vi "Handle Brushed Speed.vi"(9 "Brushless":bool, 11 "Tank Data IN":dbl[](array[numeric])) -> (3 "Tank Data OUT":dbl[](array[numeric]))   [LabVIEW 2013]
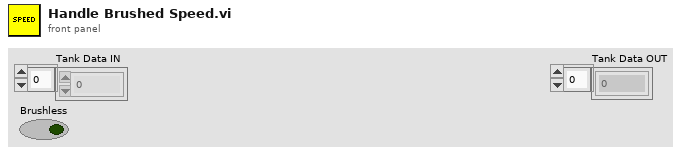
[diagram p1: front panel]
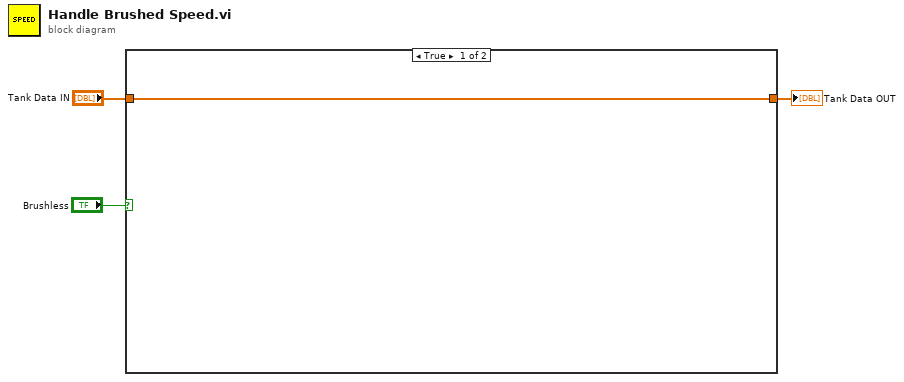
[diagram p0: block diagram]
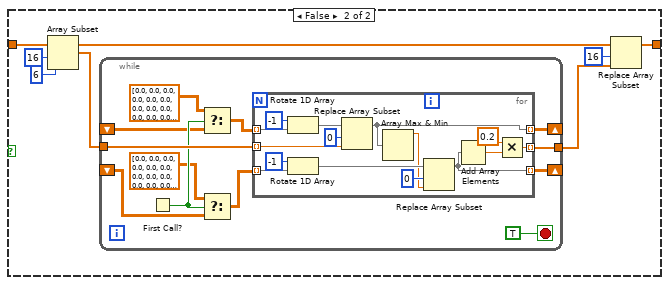
[diagram p2: hidden frame]
diagram:
  n1 = case shown="True" "Brushless" {
    tunnel: "Tank Data IN" -> [w4 w9]
    tunnel: [w4 w8] -> w2
    frame True {
    }
    frame False {
      n2 = Array Subset(array=w9, index=16, length=6 ("index")) -> (w5:dbl[])
      n3 = while {
        tunnel: [w22] -> w6
        shift-right: [w23] -> _
        shift-left: _ -> [w16]
        tunnel: w5 -> [w20]
        shift-right: [w21] -> _
        shift-left: _ -> [w17]
        stop <- TRUE stop-if-true
        n4 = First Call?() -> (First Call?: T/F=w18:bool)
        n5 = Select(t=dbl[][] [[0.0, 0.0, 0.0, 0.0, 0.0, 0.0, 0.0, 0.0, 0.0, 0.0, 0.0, 0.0, 0.0, 0.0, 0.0, 0.0, 0.0, 0.0, 0.0, 0.0], [0.0, 0.0, 0.0, 0.0, 0.0, 0.0, 0.0, 0.0, 0.0, 0.0, 0.0, 0.0, 0.0, 0.0, 0.0, 0.0, 0.0, 0.0, 0.0, 0.0], [0.0, 0.0, 0.0, 0.0, 0.0, 0.0, 0.0, 0.0, 0.0, 0.0, 0.0, 0.0, 0.0, 0.0, 0.0, 0.0, 0.0, 0.0, 0.0, 0.0], [0.0, 0.0, 0.0, 0.0, 0.0, 0.0, 0.0, 0.0, 0.0, 0.0, 0.0, 0.0, 0.0, 0.0, 0.0, 0.0, 0.0, 0.0, 0.0, 0.0], [0.0, 0.0, 0.0, 0.0, 0.0, 0.0, 0.0, 0.0, 0.0, 0.0, 0.0, 0.0, 0.0, 0.0, 0.0, 0.0, 0.0, 0.0, 0.0, 0.0], [0.0, 0.0, 0.0, 0.0, 0.0, 0.0, 0.0, 0.0, 0.0, 0.0, 0.0, 0.0, 0.0, 0.0, 0.0, 0.0, 0.0, 0.0, 0.0, 0.0]], s=w18, f=w16) -> (s? t:f=w15:dbl[][])
        n6 = Select(t=dbl[][] [[0.0, 0.0, 0.0, 0.0, 0.0], [0.0, 0.0, 0.0, 0.0, 0.0], [0.0, 0.0, 0.0, 0.0, 0.0], [0.0, 0.0, 0.0, 0.0, 0.0], [0.0, 0.0, 0.0, 0.0, 0.0], [0.0, 0.0, 0.0, 0.0, 0.0]], s=w18, f=w17) -> (s? t:f=w14:dbl[][])
        n7 = for {
          tunnel: w15 -> [w38] mode=indexing
          tunnel: w20 -> [w34] mode=indexing
          tunnel: [w33] -> w23 mode=indexing
          tunnel: [w26] -> w22 mode=indexing
          tunnel: w14 -> [w31] mode=indexing
          tunnel: [w27] -> w21 mode=indexing
          n8 = Rotate 1D Array(1:w38, 2:-1 ("n")) -> (0:w36:dbl[])
          n9 = Rotate 1D Array(1:w31, 2:-1 ("n")) -> (0:w29:dbl[])
          n10 = Replace Array Subset(array=w36, new element=w34, index=0) -> (w33:dbl[])
          n11 = Array Max & Min(array=w33) -> (max value=w28:dbl)  [unwired: 3 out]
          n12 = Replace Array Subset(array=w29, new element=w28, index=0) -> (w27:dbl[])
          n13 = Add Array Elements(numeric array=w27) -> (sum=w25:dbl)
          n14 = Multiply(x=0.2, y=w25) -> (x*y=w26:dbl)
        }
      }
      n15 = Replace Array Subset(array=w9, new element=w6, index=16) -> (w8:dbl[])
    }
  }
  "Tank Data OUT" <- w2
